vi "Set Indexer Speed.vi"(10 "Indexer backward":bool, 11 "Indexer Forward":bool) -> ()   [LabVIEW 2011]
uses:
  PID Set Points.vi
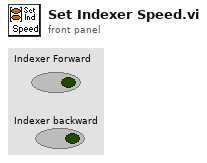
[diagram p1: front panel]
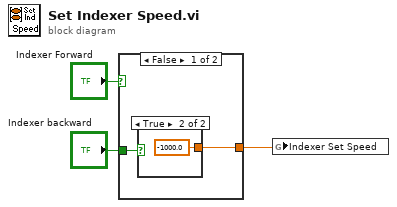
[diagram p0: block diagram]
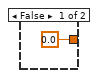
[diagram p2: hidden frame]
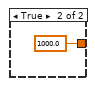
[diagram p3: hidden frame]
diagram:
  n1 = case shown="False" "Indexer Forward" {
    tunnel: [w4 1000.0] -> w1
    tunnel: "Indexer backward" -> [w5 _]
    frame False {
      n2 = case shown="True" w5 {
        tunnel: [0.0 -1000.0] -> w4
        frame False {
        }
        frame True {
        }
      }
    }
    frame True {
    }
  }
  n3 = global write "PID Set Points.vi" "Indexer Set Speed"(w1) -> ()
